vi "Keithley 2182 Relative Measurement.vi"() -> ()   [LabVIEW 2021]
doc: "Sets a reference for the specified measurement and reads a single Rel'd Measurement."
uses:
  <instrlib>/Keithley 2182/Keithley 2182.lvlib
panel:
  out "Measurement":dbl
  out "Measurement Metadata":T1
  in  "Reference Value (0)":dbl
  in  "Manually Set Reference (F: Disable)":bool
  in  "Selected Measurement Settings":T2(tab)
  in  "Voltage Resolution (8)":i32=8
  in  "Range Value (0)":dbl=10.0
  in  "Auto Range (T: Enable)":bool=TRUE
  in  "Sensor (1: Internal)":i32(ring)=1 items=["Thermocouple", "Internal"]
  in  "Reference Junction Type (0: Internal)":i32(ring) items=["Internal", "Simulated"]
  in  "Simulated Reference Temp (23 C)":dbl=23.0
  in  "Thermocouple Type (0: J)":i32(ring) items=["J", "K", "T", "E", "R", "S", "B", "N"]
  in  "Temperature Resolution (6)":i32=6
  in  "Unit (0: Celsius)":i32(ring) items=["Celsius", "Fahrenheit", "Kelvin"]
  in  "Measurement (0: Voltage Channel 1)":i32(ring) items=["Voltage Channel 1", "Voltage Channel 2", "Temperature Channel 1", "Temperature Channel 2"]
  in  "Integration Rate Units (0: Line Cycles)":i32(ring) items=["Line Cycles", "Seconds"]
  in  "Integration Rate (5)":dbl=5.0
  in  "VISA resource name":refnum<visa-resource-name>
  # "(c) 2017-2018 National Instruments.  ALL RIGHTS RESERVED."
  # "Rel'd Measurement"
  # "Measurement Settings"
  # "Step 1: Configure Measurement\nStep 2: Configure Relative Reading\nStep 3: Read Rel'd Measurement"
  # "Relative Reading Settings"
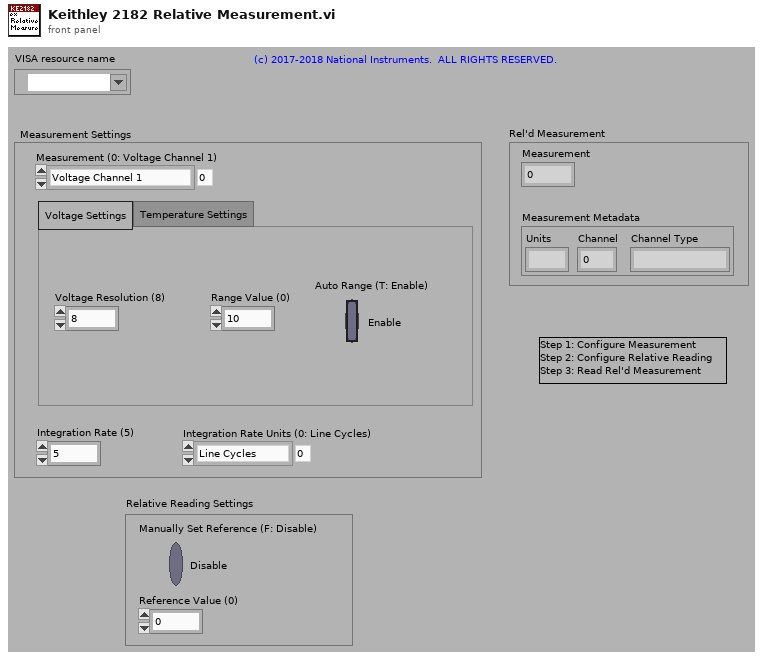
[diagram p1: front panel]
types:
  T1 = cluster{"Units":string, "Channel":i32, "Channel Type":string}
  T2 = enum32{"Voltage Settings", "Temperature Settings"}
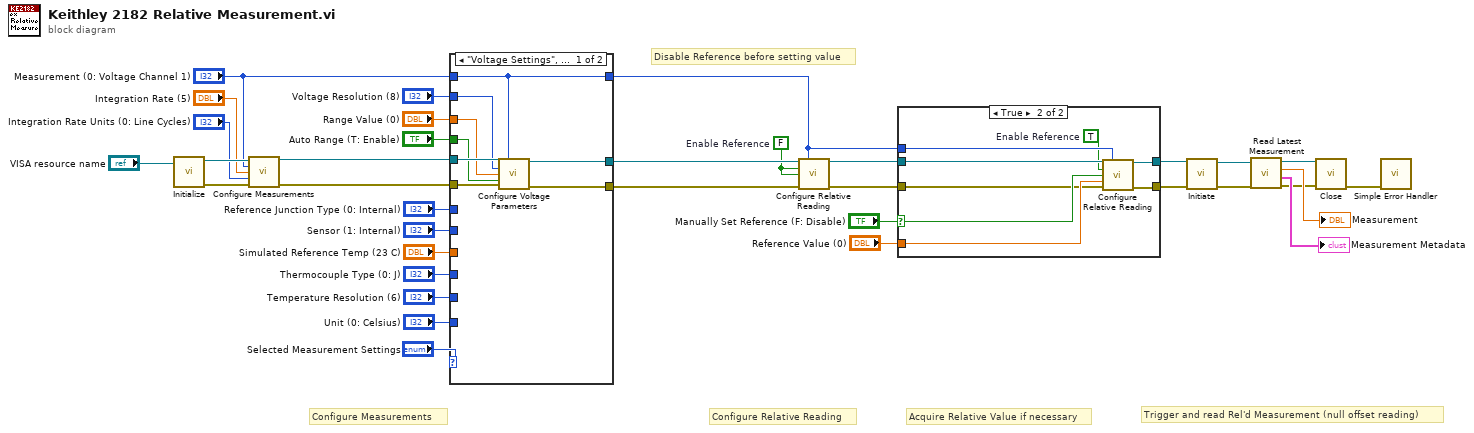
[diagram p0: block diagram]
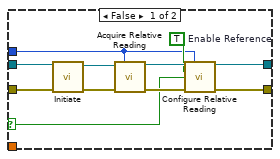
[diagram p2: hidden frame]
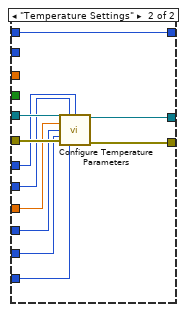
[diagram p3: hidden frame]
diagram:
  w4 = FALSE  # Enable Reference
  # "Disable Reference before setting value"
  # "Trigger and read Rel'd Measurement (null offset reading)"
  # "Acquire Relative Value if necessary"
  # "Configure Relative Reading"
  # "Configure Measurements"
  n1 = call <instrlib>:"Initialize.vi"("VISA resource name"="VISA resource name") -> ("error out"=w34:errorcluster, "VISA resource name out"=w33:refnum<visa-resource-name>)  [unwired: 9 in]
  n2 = call <instrlib>:"Configure Measurements.vi"("VISA resource name"=w33, "Measurement (0: Voltage Channel 1)"="Measurement (0: Voltage Channel 1)", "Integration Rate (5)"="Integration Rate (5)", "Integration Rate Units (0: Line Cycles)"="Integration Rate Units (0: Line Cycles)", "error in (no error)"=w34) -> ("VISA resource name out"=w27:refnum<visa-resource-name>, "error out"=w28:errorcluster)  [unwired: 9 in]
  n3 = case shown="\"Voltage Settings\", Default" "Selected Measurement Settings" {
    tunnel: "Measurement (0: Voltage Channel 1)" -> [w36 w44]
    tunnel: w28 -> [w43 w54]
    tunnel: w27 -> [w42 w51]
    tunnel: "Range Value (0)" -> [w41 _]
    tunnel: "Auto Range (T: Enable)" -> [w40 _]
    tunnel: "Voltage Resolution (8)" -> [w39 _]
    tunnel: [w38 w53] -> w17
    tunnel: [w37 w52] -> w16
    tunnel: "Unit (0: Celsius)" -> [_ w50]
    tunnel: "Reference Junction Type (0: Internal)" -> [_ w49]
    tunnel: "Sensor (1: Internal)" -> [_ w48]
    tunnel: "Simulated Reference Temp (23 C)" -> [_ w47]
    tunnel: "Thermocouple Type (0: J)" -> [_ w46]
    tunnel: "Temperature Resolution (6)" -> [_ w45]
    tunnel: [w36 w44] -> w8
    frame "Voltage Settings", Default {
      n4 = call <instrlib>:"Configure Voltage Parameters.vi"("VISA resource name"=w42, "Measurement (1: Voltage Channel 1)"=w36, "Voltage Resolution (8)"=w39, "Range Value (12)"=w41, "Autorange (T: Enable)"=w40, "error in (no error)"=w43) -> ("VISA resource name out"=w37:refnum<visa-resource-name>, "error out"=w38:errorcluster)  [unwired: 8 in]
    }
    frame "Temperature Settings" {
      n5 = call <instrlib>:"Configure Temperature Parameters.vi"("VISA resource name"=w51, "Sensor (0: Thermocouple)"=w48, "Reference Junction Type (0: Internal)"=w49, "Simulated Reference Temp (23 C)"=w47, "Thermocouple Type (0: J)"=w46, "Temperature Resolution (6)"=w45, "error in (no error)"=w54, "Unit (0: Celsius)"=w50) -> ("VISA resource name out"=w52:refnum<visa-resource-name>, "error out"=w53:errorcluster)  [unwired: 6 in]
    }
  }
  n6 = call <instrlib>:"Configure Relative Reading.vi"("VISA resource name"=w16, "Measurement (0: Voltage Channel 1)"=w8, "Enable Reference (F: Disable)"=w4, "Manually Set Reference (F: Disable)"=w4, "error in (no error)"=w17) -> ("VISA resource name out"=w13:refnum<visa-resource-name>, "error out"=w14:errorcluster)  [unwired: 9 in]
  n7 = case shown="True" "Manually Set Reference (F: Disable)" {
    selector: "Manually Set Reference (F: Disable)" -> [w57 w70]
    tunnel: w14 -> [w64 w69]
    tunnel: w13 -> [w63 w68]
    tunnel: [w59 w73] -> w6
    tunnel: [w58 w72] -> w5
    tunnel: w8 -> [w55 w67]
    tunnel: "Reference Value (0)" -> [_ w71]
    frame False {
      w56 = TRUE  # Enable Reference
      n8 = call <instrlib>:"Initiate.vi"("error in (no error)"=w64, "VISA resource name"=w63) -> ("error out"=w65:errorcluster, "VISA resource name out"=w62:refnum<visa-resource-name>)  [unwired: 8 in]
      n9 = call <instrlib>:"Acquire Relative Reading.vi"("VISA resource name"=w62, "Measurement (0: Voltage Channel 1)"=w55, "error in (no error)"=w65) -> ("VISA resource name out"=w60:refnum<visa-resource-name>, "error out"=w61:errorcluster)  [unwired: 11 in]
      n10 = call <instrlib>:"Configure Relative Reading.vi"("VISA resource name"=w60, "Measurement (0: Voltage Channel 1)"=w55, "Enable Reference (F: Disable)"=w56, "Manually Set Reference (F: Disable)"=w57, "error in (no error)"=w61) -> ("VISA resource name out"=w58:refnum<visa-resource-name>, "error out"=w59:errorcluster)  [unwired: 9 in]
    }
    frame True {
      w66 = TRUE  # Enable Reference
      n11 = call <instrlib>:"Configure Relative Reading.vi"("VISA resource name"=w68, "Measurement (0: Voltage Channel 1)"=w67, "Enable Reference (F: Disable)"=w66, "Manually Set Reference (F: Disable)"=w70, "Reference Value (0)"=w71, "error in (no error)"=w69) -> ("VISA resource name out"=w72:refnum<visa-resource-name>, "error out"=w73:errorcluster)  [unwired: 8 in]
    }
  }
  n12 = call <instrlib>:"Initiate.vi"("error in (no error)"=w6, "VISA resource name"=w5) -> ("error out"=w10:errorcluster, "VISA resource name out"=w9:refnum<visa-resource-name>)  [unwired: 8 in]
  n13 = call <instrlib>:"Read Latest Measurement.vi"("error in (no error)"=w10, "VISA resource name"=w9) -> ("error out"=w3:errorcluster, "Measurement Metadata"=→"Measurement Metadata":T1, "Measurement"=→"Measurement":dbl, "VISA resource name out"=w2:refnum<visa-resource-name>)  [unwired: 6 in]
  n14 = call <instrlib>:"Close.vi"("error in (no error)"=w3, "VISA resource name"=w2) -> ("error out"=w1:errorcluster)  [unwired: 9 in]
  n15 = call <vilib>:"Simple Error Handler.vi"("error in (no error)"=w1) -> ()  [unwired: 4 in, 5 out]
